vi "PROXY_display_single_message.vi"(8 "error_in":errorcluster, 11 "message_history_buffer_element":T1) -> (0 "error_out":errorcluster)   [LabVIEW 2020]
uses:
  FGV/DIAGNOSTICS_message_history_buffer/PROXY_DIAGNOSTICS_message_history_buffer_all_info.ctl
  STATION/station.ctl
  _misc/DIAGNOSTICS_message_type.ctl
  FGV/DIAGNOSTICS_single_message_display/FGV_PROXY_DIAGNOSTICS_single_message_display.ctl
panel:
  in  "single_message_display":i32(listbox)
  in  "STOP":bool
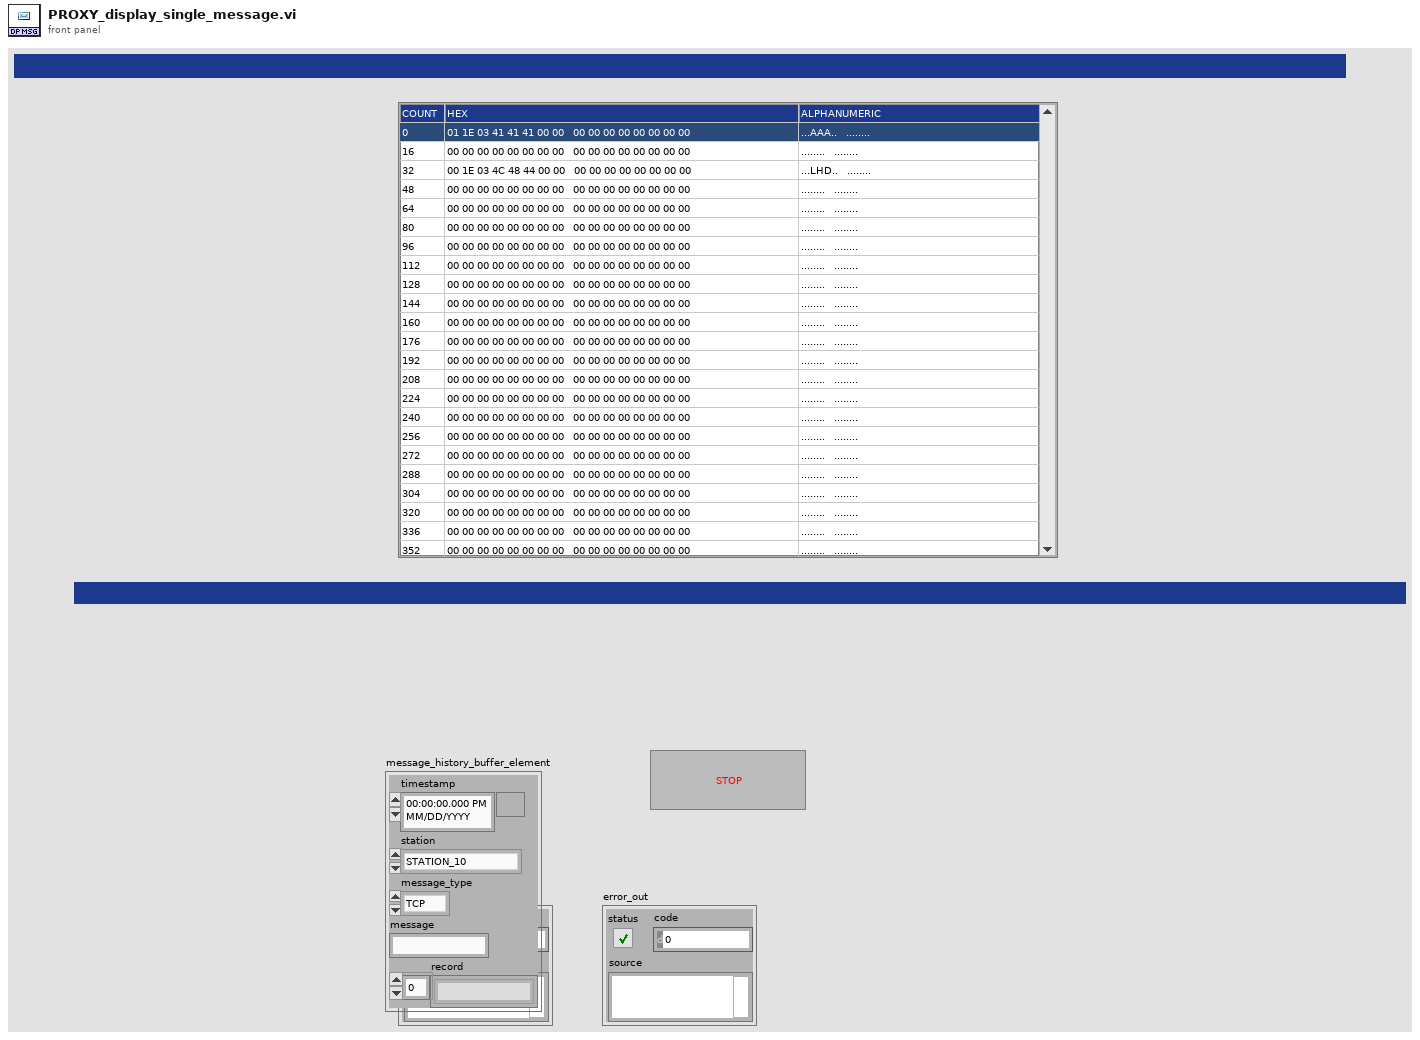
[diagram p1: front panel]
types:
  T1 = typedef "PROXY_DIAGNOSTICS_message_history_buffer_all_info.ctl" = cluster{"timestamp":timestamp, "station":T2, "message_type":T3, "message":string, "record":string[]}
  T2 = typedef "station.ctl" = enum16{"STATION_10", "STATION_20", "STATION_30", "STATION_40", "STATION_50", "STATION_60", "STATION_70", "STATION_80", "STATION_90", "STATION_100", "STATION_110", "STATION_120", "STATION_165", "MAIN"}
  T3 = typedef "DIAGNOSTICS_message_type.ctl" = enum16{"TCP", "SQL"}
  T4 = typedef "FGV_PROXY_DIAGNOSTICS_single_message_display.ctl" = enum16{"initialize", "display_message"}
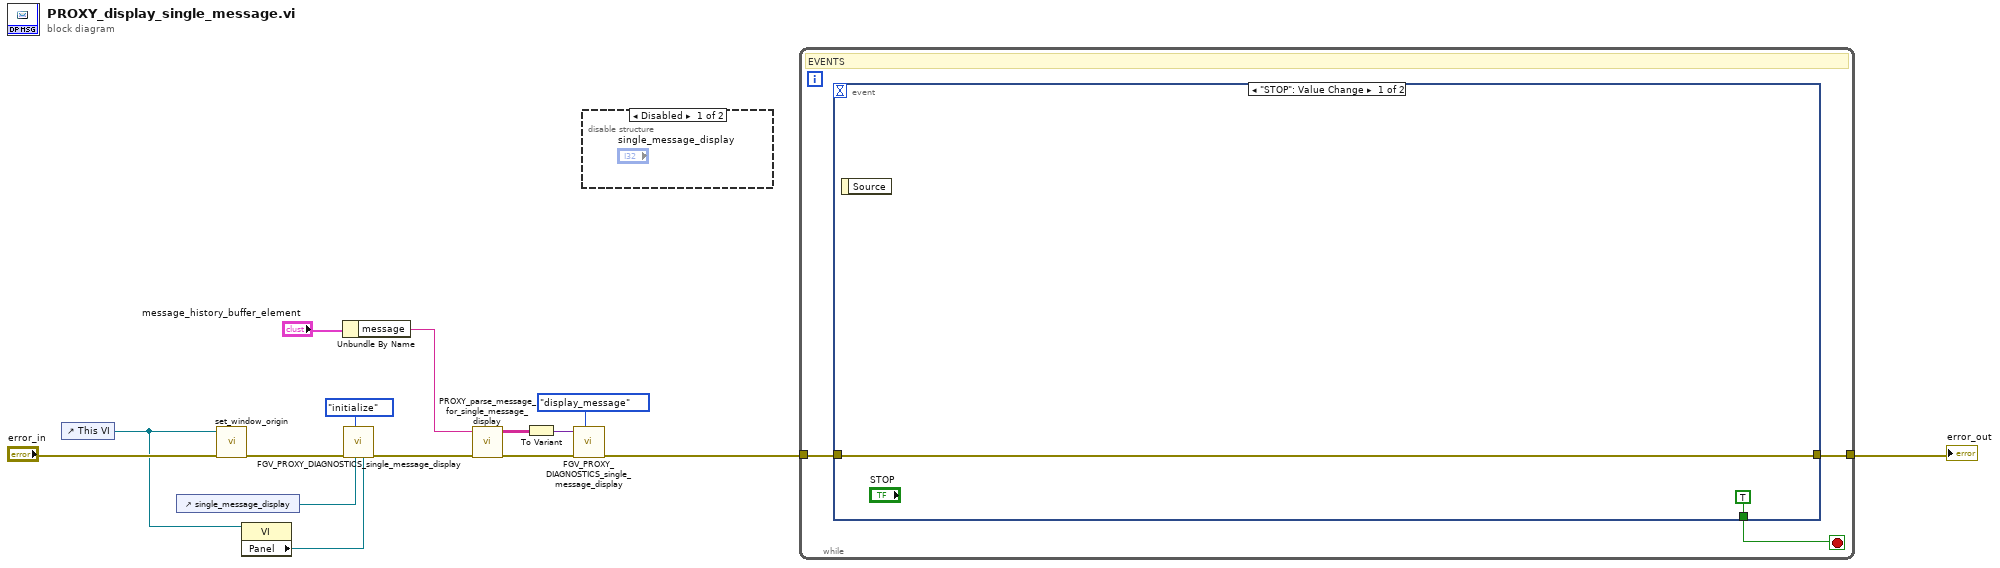
[diagram p0: block diagram]
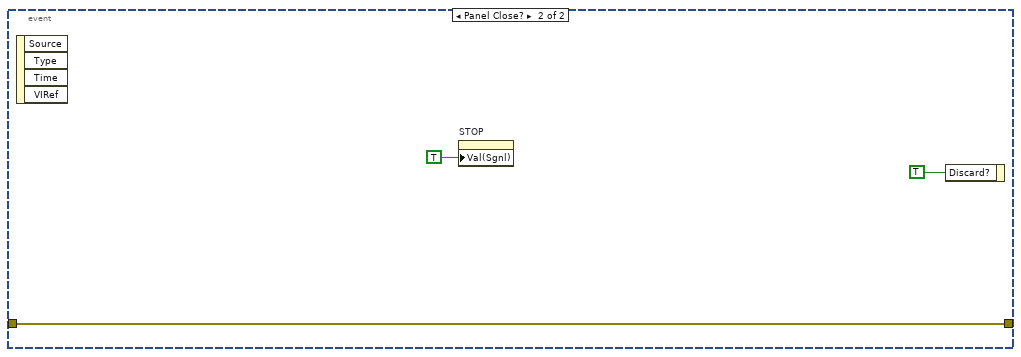
[diagram p3: hidden frame]
diagram:
  n1 = control-ref of="This VI"() -> (w8:refnum<vi>)
  n2 = control-ref of="single_message_display"() -> (w10:refnum<vi>)
  n3 = call "set_window_origin.vi"("error_in"="error_in", "this_vi_reference"=w8) -> ("error_out"=w11:errorcluster)  [unwired: 9 in]
  n4 = property class="VI"(reference=w8) -> ("Panel"=w9:refnum<vi>)  [unwired: 1 in, 2 out]
  n5 = Unbundle By Name("message_history_buffer_element") -> ("message"=w12:string)
  n6 = call "FGV_PROXY_DIAGNOSTICS_single_message_display.vi"("front_panel_reference"=w9, "SQL_listbox_reference"=w10, "options"=FGV_PROXY_DIAGNOSTICS_single_message_display."initialize", "error_in"=w11) -> ("error_out"=w5:errorcluster)  [unwired: 7 in]
  n7 = call "PROXY_parse_message_for_single_message_display.vi"("error_in"=w5, "message"=w12) -> ("error_out"=w4:errorcluster, "parsed_message"=w2:string[][])  [unwired: 8 in]
  n8 = To Variant(anything=w2) -> (Variant=w3:variant)
  n9 = call "FGV_PROXY_DIAGNOSTICS_single_message_display.vi"("options"=FGV_PROXY_DIAGNOSTICS_single_message_display."display_message", "error_in"=w4, "input"=w3) -> ("error_out"=w1:errorcluster)  [unwired: 8 in]
  n10 = disable-structure shown="Disabled" {
    frame Disabled {
    }
    frame Enabled {
    }
  }
  n11 = while {
    tunnel: [w18] -> w15
    tunnel: w1 -> [w16]
    stop <- w17 stop-if-true
    # "EVENTS"
    n12 = event shown="[0] \"STOP\": Value Change" {
      selector: _ -> [_ _]
      dyn-events: _ -> [_ _]
      timeout: _ -> [_ _]
      tunnel: [TRUE _] -> w17
      tunnel: w16 -> [w20 w23]
      tunnel: [w20 w23] -> w18
      event "STOP": Value Change {
        n13 = event-data() -> ()  [unwired: 1 in, 1 out]
      }
      event Panel Close? {
        n14 = event-data() -> ()  [unwired: 1 in, 4 out]
        n15 = property on="STOP" class="Bool (strict)"("Val(Sgnl)"=TRUE ("Value (Signaling)")) -> ()  [unwired: 2 in, 2 out]
        n16 = event-data("Discard?"=TRUE) -> ()  [unwired: 1 in, 1 out]
      }
    }
  }
  "error_out" <- w15
